vi "Auto_Routine_DepositHighBackup.vi"(8 "error in (no error)":errorcluster) -> (0 "error out":errorcluster)   [LabVIEW 2020]
doc: "Deposits a cone on the upper node then backs up\nInputs: \n--ErrorIn--\nOutputs:\n--ErrorOut--"
uses:
  Arm/ArmPositionPreset.ctl
  Arm/ArmGamePiecePreset.ctl
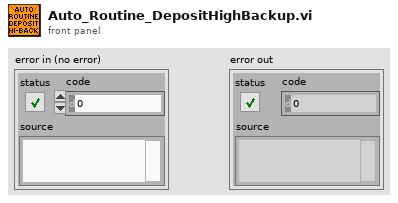
[diagram p1: front panel]
types:
  T1 = typedef "ArmGamePiecePreset.ctl" = enum16{"Cube", "Cone"}
  T2 = typedef "ArmPositionPreset.ctl" = enum16{"Upper", "Lower", "Middle", "Home", "Shelf", "Floor", "HalfFloor", "HalfHome"}
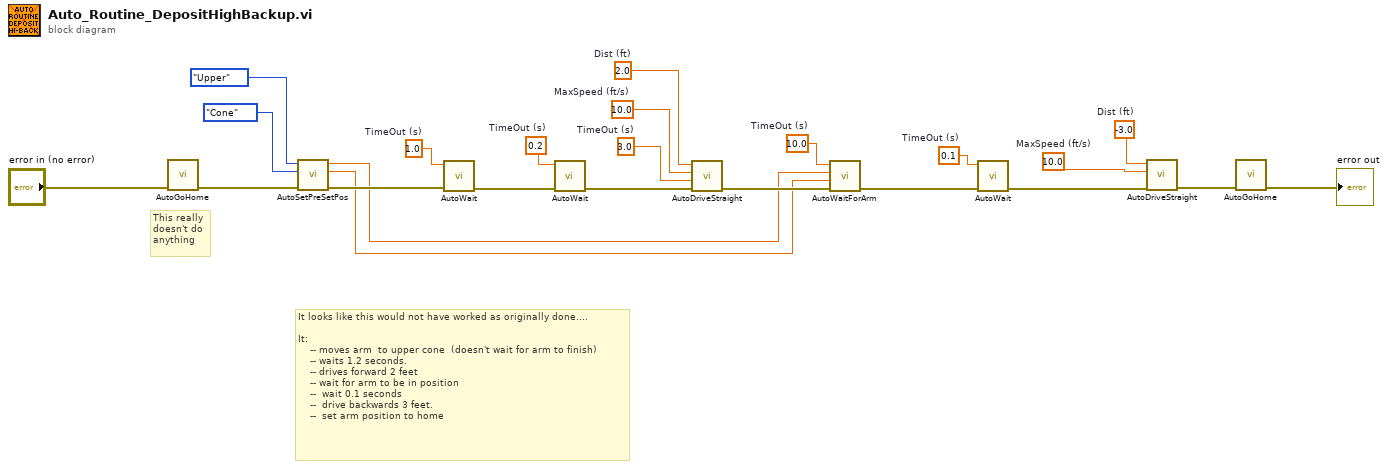
[diagram p0: block diagram]
diagram:
  w23 = 1.0  # TimeOut (s)
  w21 = 10.0  # MaxSpeed (ft/s)
  w20 = 3.0  # TimeOut (s)
  w19 = 10.0  # MaxSpeed (ft/s)
  w18 = 2.0  # Dist (ft)
  w16 = -3.0  # Dist (ft)
  w15 = 0.1  # TimeOut (s)
  w14 = 0.2  # TimeOut (s)
  w13 = 10.0  # TimeOut (s)
  # "This really\ndoesn't do\nanything"
  # "It looks like this would not have worked as originally done....\n\nIt:\n    -- moves arm  to upper cone  (doesn't wait for arm to finish)\n    -- waits 1.2 seconds.\n    -- drives forward 2 feet\n    -- wait for arm to be in position\n    --  wait 0.1 seconds\n    --  drive backwards 3 feet.\n    --  set arm position to home"
  n1 = call "AutoGoHome.vi"("error in (no error)"="error in (no error)") -> ("error out"=w6:errorcluster)  [unwired: 8 in, 2 out]
  n2 = call "AutoSetPreSetPos.vi"("error in (no error)"=w6, "Game Piece"=ArmGamePiecePreset."Cone", "Position"=ArmPositionPreset."Upper") -> ("error out"=w22:errorcluster, "Desired Extend"=w1:dbl, "Desired Lift"=w2:dbl)  [unwired: 6 in]
  n3 = call "AutoWait.vi"("error in (no error)"=w22, "TimeOut (s)"=w23) -> ("error out"=w7:errorcluster)  [unwired: 9 in]
  n4 = call "AutoWait.vi"("error in (no error)"=w7, "TimeOut (s)"=w14) -> ("error out"=w11:errorcluster)  [unwired: 9 in]
  n5 = call "AutoDriveStraight.vi"("error in (no error)"=w11, "TimeOut (s)"=w20, "MaxSpeed (ft/s)"=w19, "Dist (ft)"=w18) -> ("error out"=w12:errorcluster)  [unwired: 7 in]
  n6 = call "AutoWaitForArm.vi"("error in (no error)"=w12, "Desired Extend"=w1, "Desired Lift"=w2, "TimeOut (s)"=w13) -> ("error out"=w5:errorcluster)  [unwired: 7 in]
  n7 = call "AutoWait.vi"("error in (no error)"=w5, "TimeOut (s)"=w15) -> ("error out"=w17:errorcluster)  [unwired: 9 in]
  n8 = call "AutoDriveStraight.vi"("error in (no error)"=w17, "MaxSpeed (ft/s)"=w21, "Dist (ft)"=w16) -> ("error out"=w8:errorcluster)  [unwired: 8 in]
  n9 = call "AutoGoHome.vi"("error in (no error)"=w8) -> ("error out"=→"error out":errorcluster)  [unwired: 8 in, 2 out]
